vi "AR_Basic.vi"   [LabVIEW 2012]
types:
  T1 = typedef "BotSpeak_Control.ctl" = cluster{"Address":string, "Reply EOF":string, "Hardware":string, "Retries":i8, "Timeout":i32}
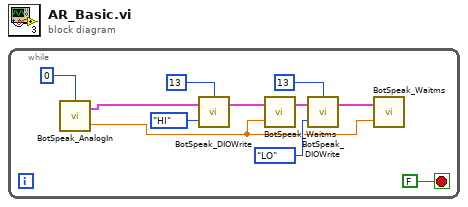
[diagram p0: block diagram]
diagram:
  n1 = while {
    stop <- FALSE stop-if-true
    n2 = call <userlib>:"BotSpeak_AnalogIn.vi"("A/D Channel"=u8 0) -> ("voltage"=w3:dbl, "Bot Settings"=w2:T1)  [unwired: 2 in]
    n3 = call <userlib>:"BotSpeak_DIOWrite.vi"("State"=enum32{"LO", "HI"}."HI", "Bot Settings"=w2, "DIO Line"=u32 13) -> ("Bot Settings"=w9:T1)  [unwired: 1 out]
    n4 = call <userlib>:"BotSpeak_Waitms.vi"("Wait (ms)"=w3, "Bot Settings"=w9) -> ("Bot Settings 2"=w8:T1)  [unwired: 1 in]
    n5 = call <userlib>:"BotSpeak_DIOWrite.vi"("State"=enum32{"LO", "HI"}."LO", "Bot Settings"=w8, "DIO Line"=u32 13) -> ("Bot Settings"=w7:T1)  [unwired: 1 out]
    n6 = call <userlib>:"BotSpeak_Waitms.vi"("Wait (ms)"=w3, "Bot Settings"=w7) -> ()  [unwired: 1 in, 1 out]
  }
